vi "MassFlowRate_ExpFactor.vi"(9 "Differential Pressure":dbl(knob) scale=0.0..2.0, 10 "Upstream Pressure":dbl(knob) scale=0.0..300.0, 11 "Upstream \nTemperature":dbl(slide) scale=0.0..40.0) -> (3 "Mass Flow Rate":dbl)   [LabVIEW 2022 SP3]
panel:
  out "Upstream Density":dbl
  out "Beta":dbl
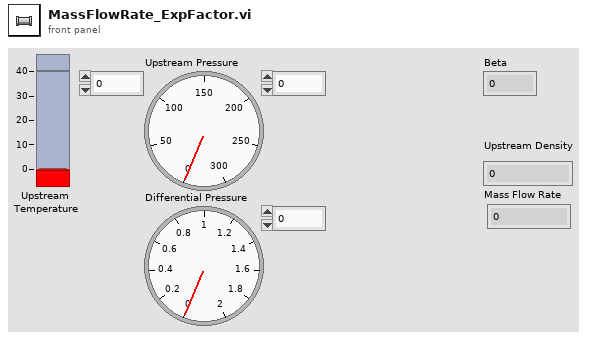
[diagram p1: front panel]
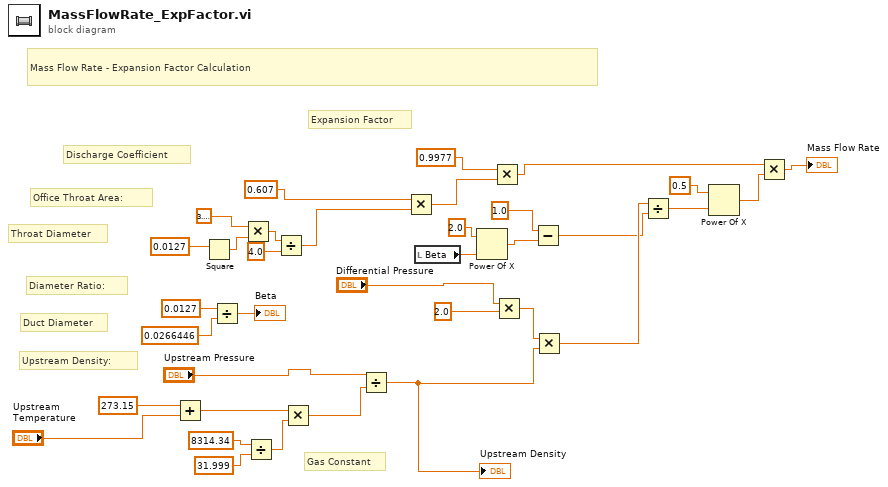
[diagram p0: block diagram]
diagram:
  # "Expansion Factor"
  # "Mass Flow Rate - Expansion Factor Calculation"
  # "Gas Constant"
  # "Upstream Density:"
  # "Duct Diameter"
  # "Diameter Ratio:"
  # "Discharge Coefficient"
  # "Office Throat Area:"
  # "Throat Diameter"
  n1 = Add(x=273.15, y="Upstream \nTemperature") -> (x+y=w22:dbl)
  n2 = Square(x=0.0127) -> (x^2=w33:dbl)
  n3 = Divide(x=0.0127, y=0.0266446 ("x")) -> (x/y=→"Beta":dbl)
  n4 = Multiply(x=3.141592653589793, y=w33) -> (x*y=w32:dbl)
  n5 = Divide(x=8314.34, y=31.999 ("x")) -> (x/y=w21:dbl)
  n6 = Divide(x=w32, y=4.0) -> (x/y=w30:dbl)
  n7 = Multiply(x=w22, y=w21) -> (x*y=w20:dbl)
  n8 = Divide(x="Upstream Pressure", y=w20) -> (x/y=w17:dbl)
  "Upstream Density" <- w17
  n9 = Multiply(x=0.607, y=w30) -> (x*y=w7:dbl)
  n10 = local read "Beta"() -> (w14:dbl)
  n11 = Power Of X(1:w14, 2:2.0 ("y")) -> (0:w13:dbl)
  n12 = Multiply(x=0.9977, y=w7) -> (x*y=w5:dbl)
  n13 = Multiply(x="Differential Pressure", y=2.0) -> (x*y=w18:dbl)
  n14 = Subtract(x=1.0, y=w13) -> (x-y=w11:dbl)
  n15 = Multiply(x=w18, y=w17) -> (x*y=w16:dbl)
  n16 = Divide(x=w16, y=w11) -> (x/y=w10:dbl)
  n17 = Power Of X(1:w10, 2:0.5) -> (0:w8:dbl)
  n18 = Multiply(x=w5, y=w8) -> (x*y=→"Mass Flow Rate":dbl)
